vi "Update inventary.vi"(8 "error in (no error)":errorcluster, 9 "Indice":i32, 10 "Inventario":dbl, 11 "Nestle Actor in":refnum<class "Nestle Actor.lvclass">) -> (0 "error out":errorcluster, 3 "Nestle Actor out":refnum<class "Nestle Actor.lvclass">)   [LabVIEW 2020, in "Nestle Actor.lvlib" / "Nestle Actor.lvclass"]
uses:
  Nestle Actor.lvclass
  Nestle Actor.lvclass/Nestle Actor.ctl
  <vilib>/Utility/config.llb/Write Key (String).vi
  <vilib>/Utility/config.llb/NI_LVConfig.lvlib
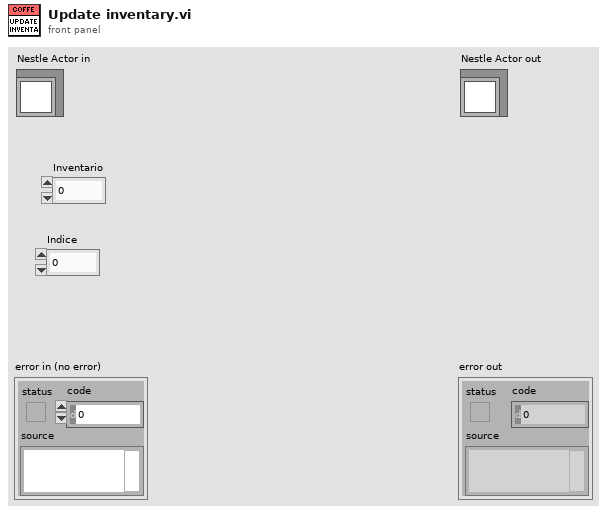
[diagram p1: front panel]
types:
  T1 = typedef "NI_LVConfig.lvlib/Config Data RefNum.ctl" = refnum<k1>
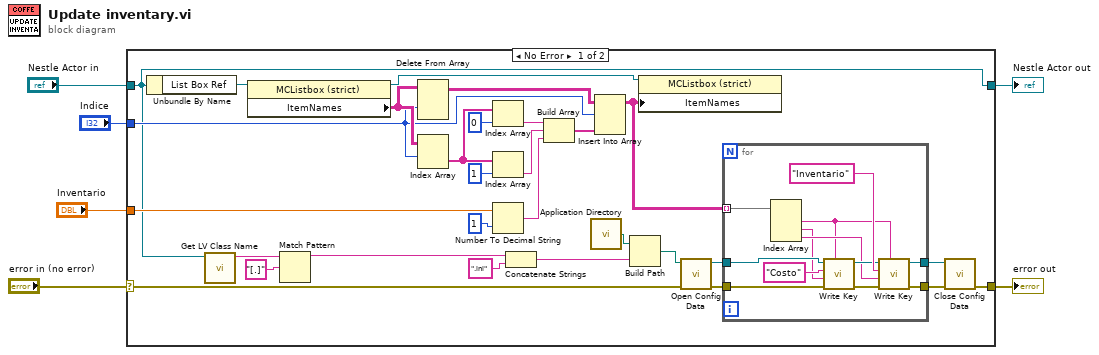
[diagram p0: block diagram]
diagram:
  n1 = case shown="No Error" "error in (no error)" {
    selector: "error in (no error)" -> [w9 w49]
    tunnel: [w8 w49] -> w5
    tunnel: [w7 w48] -> w3
    tunnel: "Nestle Actor in" -> [w7 w48]
    tunnel: "Indice" -> [w11 _]
    tunnel: "Inventario" -> [w10 _]
    frame No Error {
      n2 = Unbundle By Name(w7) -> ("List Box Ref"=w35:refnum<vi>)
      n3 = call <vilib>:"Get LV Class Name.vi"("object"=w7) -> ("class name"=w28:string)  [unwired: 9 in, 1 out]
      n4 = property class="MCListbox (strict)"(reference=w35) -> (reference out=w12:refnum<vi>, "ItemNames"=w16:string[][])  [unwired: 1 in, 1 out]
      n5 = Match Pattern(string=w28, regular expression="[.]") -> (before substring=w29:string)  [unwired: 1 in, 3 out]
      n6 = Delete From Array(array=w16, index (row)=w11) -> (array with subset deleted=w15:string[][])  [unwired: 2 in, 1 out]
      n7 = Index Array(array=w16, index (row)=w11) -> (element=w25:string[])  [unwired: 1 in]
      n8 = Index Array(array=w25, index=0) -> (element=w24:string)
      n9 = Index Array(array=w25, index=1) -> (element=w23:string)
      n10 = Number To Decimal String(number=w10, width (-)=i16 1) -> (decimal integer string=w22:string)
      n11 = Concatenate Strings(w29, ".ini") -> (w33:string)
      n12 = Build Array(w24, w23, w22) -> (w14:string[])
      n13 = call <vilib>:"Application Directory.vi"() -> ("Application Directory"=w34:path)
      n14 = Insert Into Array(array=w15, index (row)=w11, new element=w14) -> (w13:string[][])  [unwired: 1 in]
      n15 = Build Path(base path=w34, name or relative path=w33) -> (appended path=w31:path)
      n16 = property class="MCListbox (strict)"(reference=w12, "ItemNames"=w13) -> ()  [unwired: 1 in, 2 out]
      n17 = call <vilib>:"Open Config Data.vi"("error in (no error)"=w9, "configuration file path"=w31) -> ("error out"=w19:errorcluster, "refnum"=w20:T1)  [unwired: 7 in, 1 out]
      n18 = for {
        tunnel: w20 -> [w45]
        tunnel: w19 -> [w44]
        tunnel: [w41] -> w18
        tunnel: [w40] -> w17
        tunnel: w13 -> [w39] mode=indexing
        n19 = Index Array(array=w39) -> (element #1=w37:string, element #2=w36:string, element #3=w38:string)  [unwired: 3 in]
        n20 = call-poly <vilib>:"Write Key.vi"("section"=w37, "error in (no error)"=w44, "value"=w36, "key"="Costo", "refnum"=w45) -> ("error out"=w42:errorcluster, "refnum out"=w43:T1)  [unwired: 4 in, 1 out]
        n21 = call-poly <vilib>:"Write Key.vi"("section"=w37, "error in (no error)"=w42, "value"=w38, "key"="Inventario", "refnum"=w43) -> ("error out"=w40:errorcluster, "refnum out"=w41:T1)  [unwired: 4 in, 1 out]
      }
      n22 = call <vilib>:"Close Config Data.vi"("error in (no error)"=w17, "refnum"=w18) -> ("error out"=w8:errorcluster)  [unwired: 8 in, 1 out]
    }
    frame Error {
    }
  }
  "error out" <- w5
  "Nestle Actor out" <- w3
